vi "Handshake RFC6455.vi"(0 "websocket client handshake":string="GET / HTTP/1.1\r\nUpgrade: websocket\r\nConnection: Upgrade\r\nHost: localhost:81\r\nOrigin: null\r\nSec-WebSocket-Key: dGhlIHNhbXBsZSBub25jZQ==\r\nSec-WebSocket-Version: 13\r\n\r\n") -> (1 "accept string":string, 2 "websocket server handshake":string)   [LabVIEW 2014, in "FrontPanelPublisher.lvlib" / "Websocket.lvclass"]
uses:
  Websocket.lvclass
  Common/SHA-1 Digest.vi
  Common/SHA-1 Core.vi
  Common/SHA-1 Pad.vi
  FrontPanelPublisher.lvlib
panel:
  out "hash string":string
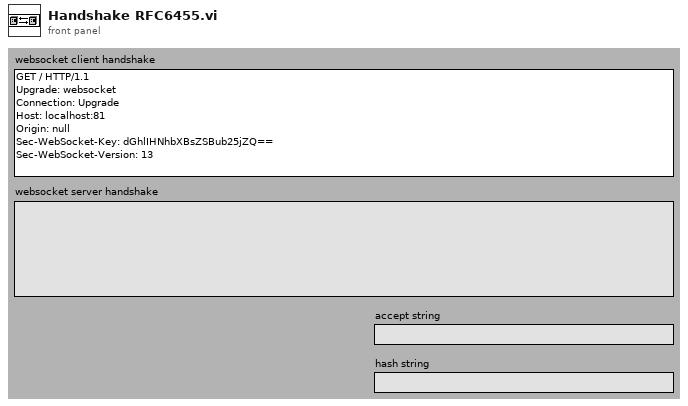
[diagram p1: front panel]
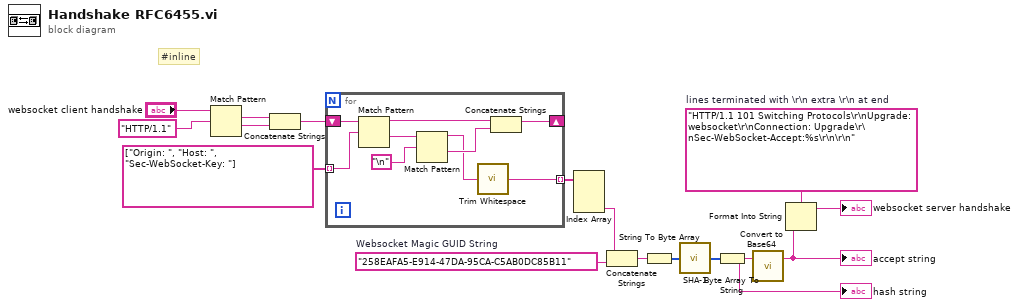
[diagram p0: block diagram]
diagram:
  w1 = "HTTP/1.1 101 Switching Protocols\r\nUpgrade: websocket\r\nConnection: Upgrade\r\nSec-WebSocket-Accept:%s\r\n\r\n"  # lines terminated with \r\n extra \r\n at end
  w7 = "258EAFA5-E914-47DA-95CA-C5AB0DC85B11"  # Websocket Magic GUID String
  # "#inline"
  n1 = Match Pattern(string="websocket client handshake", regular expression="HTTP/1.1") -> (match substring=w10:string, after substring=w15:string)  [unwired: 1 in, 2 out]
  n2 = Concatenate Strings(w10, w15) -> (w14:string)
  n3 = for {
    shift-right: [w21] -> _
    shift-left: w14 -> [w25]
    tunnel: [w17] -> w12 mode=indexing
    tunnel: string[] ["Origin: ", "Host: ", "Sec-WebSocket-Key: "] -> [w19] mode=indexing
    n4 = Match Pattern(string=w25, regular expression=w19) -> (before substring=w23:string, after substring=w24:string)  [unwired: 1 in, 2 out]
    n5 = Match Pattern(string=w24, regular expression="\n") -> (before substring=w20:string, after substring=w22:string)  [unwired: 1 in, 2 out]
    n6 = call <vilib>:"Trim Whitespace.vi"("string"=w20) -> ("trimmed string"=w17:string)  [unwired: 1 in]
    n7 = Concatenate Strings(w23, w22) -> (w21:string)
  }
  n8 = Index Array(array=w12) -> (element #3=w8:string)  [unwired: 3 in, 2 out]
  n9 = Concatenate Strings(w8, w7) -> (w6:string)
  n10 = String To Byte Array(string=w6) -> (unsigned byte array=w5:u8[])
  n11 = call "SHA-1.vi"("Data"=w5) -> ("message-digest"=w4:u8[])
  n12 = Byte Array To String(unsigned byte array=w4) -> (string=w3:string)
  "hash string" <- w3
  n13 = call "Convert to Base64.vi"("String"=w3) -> ("Base64 String"=w2:string)  [unwired: 2 in]
  "accept string" <- w2
  n14 = Format Into String(format string=w1, w2) -> (resulting string=→"websocket server handshake":string)  [unwired: 2 in, 1 out]
